vi "Drive Controller.vi"(8 "error in":errorcluster) -> ()   [LabVIEW 2023]
doc: "This VI executes continuously carrying out the current operation and responding to updates or new operation requests. It will often contain the timing or control code that is difficult to place directly in TeleOp. This VI generally opens all sensors and motors and isolates the rest of the robot code from knowing implementation details of how the operations are carried out."
uses:
  Drive Setpoints.ctl
  Drive Operations.ctl
  swerve-template/Type Definitions/Data/Robot Velocities.ctl
  <vilib>/Rock Robotics/WPI/ThirdParty/REV Robotics/REVLib/Typedef/Spark MAX Control Type.ctl
  80b923c8-6b82-42f9-a8cd-acddf0fa8107.vi
  Framework/Robot Global Data.vi
panel:
  in  "Drive Controller Diagnostics":T1(tab)
  out "Swerve Visualizer":cluster{dbl[], dbl[]}[](graph)
  out "Pod Comparisons (Diff -> Setpoint - Actual)":T2
  out "(Calibration) Steering Angles":T3
  out "Current\nCmd":string
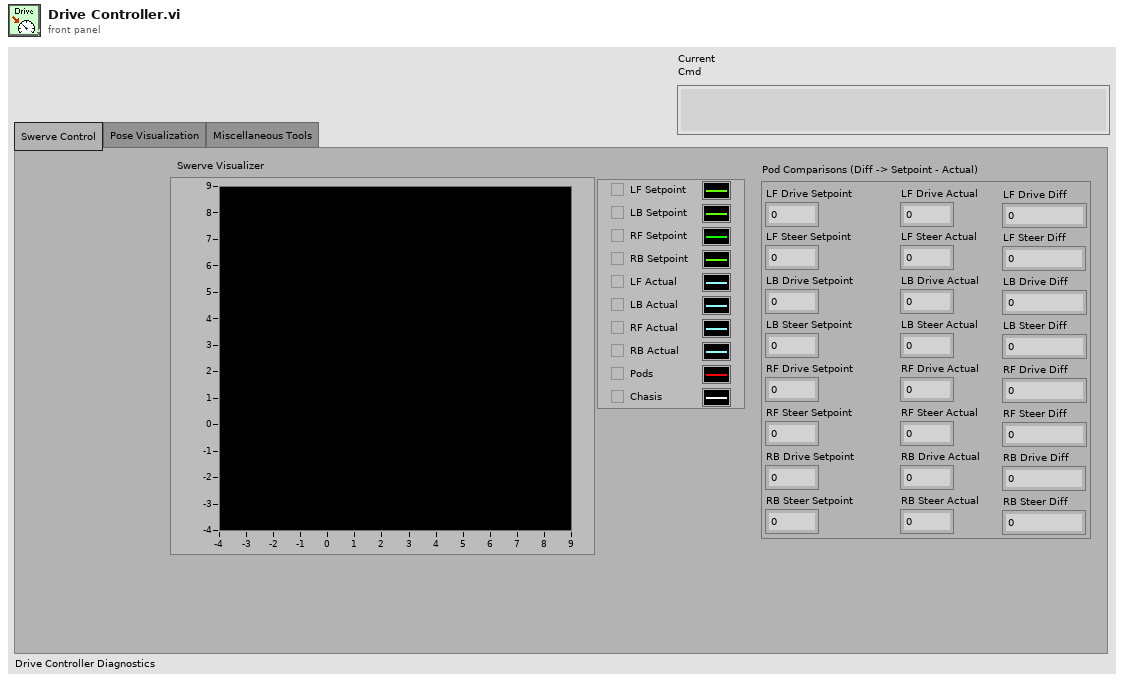
[diagram p1: front panel]
types:
  T1 = enum32{"Swerve Control", "Pose Visualization", "Miscellaneous Tools"}
  T2 = cluster{"LF Drive Setpoint":dbl, "LF Steer Setpoint":dbl, "LB Drive Setpoint":dbl, "LB Steer Setpoint":dbl, "RF Drive Setpoint":dbl, "RF Steer Setpoint":dbl, "RB Drive Setpoint":dbl, "RB Steer Setpoint":dbl, "LF Drive Actual":dbl, "LF Steer Actual":dbl, "LB Drive Actual":dbl, "LB Steer Actual":dbl, "RF Drive Actual":dbl, "RF Steer Actual":dbl, "RB Drive Actual":dbl, "RB Steer Actual":dbl, "LF Drive Diff":dbl, "LF Steer Diff":dbl, "LB Drive Diff":dbl, "LB Steer Diff":dbl, "RF Drive Diff":dbl, "RF Steer Diff":dbl, "RB Drive Diff":dbl, "RB Steer Diff":dbl}
  T3 = cluster{"Left Front":dbl, "Left Back":dbl, "Right Front":dbl, "Right Back":dbl}
  T4 = typedef "Drive Setpoints.ctl" = cluster{"Operation":T5, "Robot Velocities":T6, "Auto Data":cluster{"Auto Velocities":T6[], "Auto Positions":cluster{"x":dbl, "y":dbl, "th":dbl}[], "Auto Commands":cluster{dbl, "Command out":cluster{"Name":string, "vi reference":refnum<vi>, i32[], variant[]}}[], "Zero Velocity?":bool[]}}
  T5 = typedef "Drive Operations.ctl" = enum16{"Reserve", "Read Current", "Immediate", "Calibrate", "Auto"}
  T6 = typedef "Robot Velocities.ctl" = cluster{"X Velocity":dbl, "Y Velocity":dbl, "Rotational \nVelocity":dbl}
  T7 = typedef "(NEO-NEO-ThroughBore-Pigeon2) Swerve.ctl" = cluster{"Drive Motors (NEO)":T8, "Steer Motors (NEO)":T8, "Pigeon2":T14, "Radii (ft)":T16}
  T8 = typedef "(NEO & NEO 550) 4 Motor Set.ctl" = cluster{"Left Front":T9, "Left Back":T9, "Right Front":T9, "Right Back":T9}
  T9 = typedef "WPI_MotorControlDeviceRef.ctl" = cluster{"DeviceStatus":errorcluster, "Type":T10, "PWM":cluster{"PWM Channel":T11, "DeadBand":T12}, "CAN":cluster{"Device Number":u8, "SetOutput VI Ref":variant, "GetOutput VI Ref":variant, "Enable VI Ref":variant, "Disable VI Ref":variant, "Data":variant}, "Invert":bool, "DIO PWM":cluster{"PWM \"Enable\" Channel":T11, "DIOChannel":T13, "PWM Rate":dbl}}
  T10 = typedef "WPI_MotorControlType.ctl" = enum16{"PWM", "CAN", "DIO PWM"}
  T11 = typedef "FPGA_DIOPWMChannel.ctl" = enum8{"PWM 0", "PWM 1", "PWM 2", "PWM 3", "PWM 4", "PWM 5", "PWM 6", "PWM 7", "PWM 8", "PWM 9", "PWM MXP 0", "PWM MXP 1", "PWM MXP 2", "PWM MXP 3", "PWM MXP 4", "PWM MXP 5", "PWM MXP 6", "PWM MXP 7", "PWM MXP 8", "PWM MXP 9", "Invalid"}
  T12 = typedef "WPI_PWMDeadband.ctl" = cluster{"Name":string, "maxPositivePwm":i32, "minPositivePwm":i32, "centerPwm":i32, "maxNegativePwm":i32, "minNegativePwm":i32, "angularRange":u16}
  T13 = typedef "FPGA_DIOChannel.ctl" = enum8{"DIO 0", "DIO 1", "DIO 2", "DIO 3", "DIO 4", "DIO 5", "DIO 6", "DIO 7", "DIO 8", "DIO 9", "DIO MXP 0", "DIO MXP 1", "DIO MXP 2", "DIO MXP 3", "DIO MXP 4", "DIO MXP 5", "DIO MXP 6", "DIO MXP 7", "DIO MXP 8", "DIO MXP 9", "DIO MXP 10", "DIO MXP 11", "DIO MXP 12", "DIO MXP 13", "DIO MXP 14", "DIO MXP 15", "SPI Port CS1", "SPI Port CS2", "SPI Port CS3", "SPI Port MISO", "SPI Port MOSI", "Invalid"}
  T14 = typedef "CTRE_PigeonIMU_DeviceRef.ctl" = cluster{"DeviceStatus":errorcluster, "Device Number":u8, "Type":T15, "Device ID":u32, "Handle":u64, "UsageFrame":u32, "Library Path":path}
  T15 = typedef "CTRE_PigeonIMU_ConnectionType.ctl" = u32
  T16 = typedef "Pod Positions.ctl" = cluster{"Left Front Position":dbl[], "Left Back Position":dbl[], "Right Front Position":dbl[], "Right Back Position":dbl[]}
  T17 = typedef "Command Status Info.ctl" = cluster{"Name":string, "Status":T18, "notifier out":T19}
  T18 = typedef "Completion Status.ctl" = enum16{"Successful", "Aborted", "Incomplete"}
  T19 = typedef "Completion Notifier.ctl" = refnum<notifier>
  T20 = cluster{"SubSystem Data":T4, cluster{"Start Time (ms)":u32, "Iterations":i32}, cluster{"Command Info":T17, "Description":string, "Default Command":T4, "queue out":refnum<queue>, "Subsystem Name":string}}
  T21 = cluster{"Auto Velocities":T6[], "Auto Positions":cluster{"x":dbl, "y":dbl, "th":dbl}[], "Auto Commands":cluster{dbl, "Command out":cluster{"Name":string, "vi reference":refnum<vi>, i32[], variant[]}}[], "Zero Velocity?":bool[]}
  T22 = typedef "Pod Setpoints.ctl" = cluster{"Left Front":cluster{"Velocity":dbl, "Theta":dbl}, "Left Back":cluster{"Velocity":dbl, "Theta":dbl}, "Right Front":cluster{"Velocity":dbl, "Theta":dbl}, "Right Back":cluster{"Velocity":dbl, "Theta":dbl}}
  T23 = typedef "Spark MAX Control Type.ctl" = enum16{"Percent VBus", "Voltage", "Velocity", "Position", "Smart Motion", "Current", "Smart Velocity", "MAXMotion Position", "MAXMotion Velocity"}
  T24 = cluster{"SubSystem Data":T4, cluster{"Start Time (ms)":u32, "Iterations":i32}, "Default Command Arguments":cluster{"Command Info":T17, "Description":string, "Default Command":T4, "queue out":refnum<queue>, "Subsystem Name":string}}
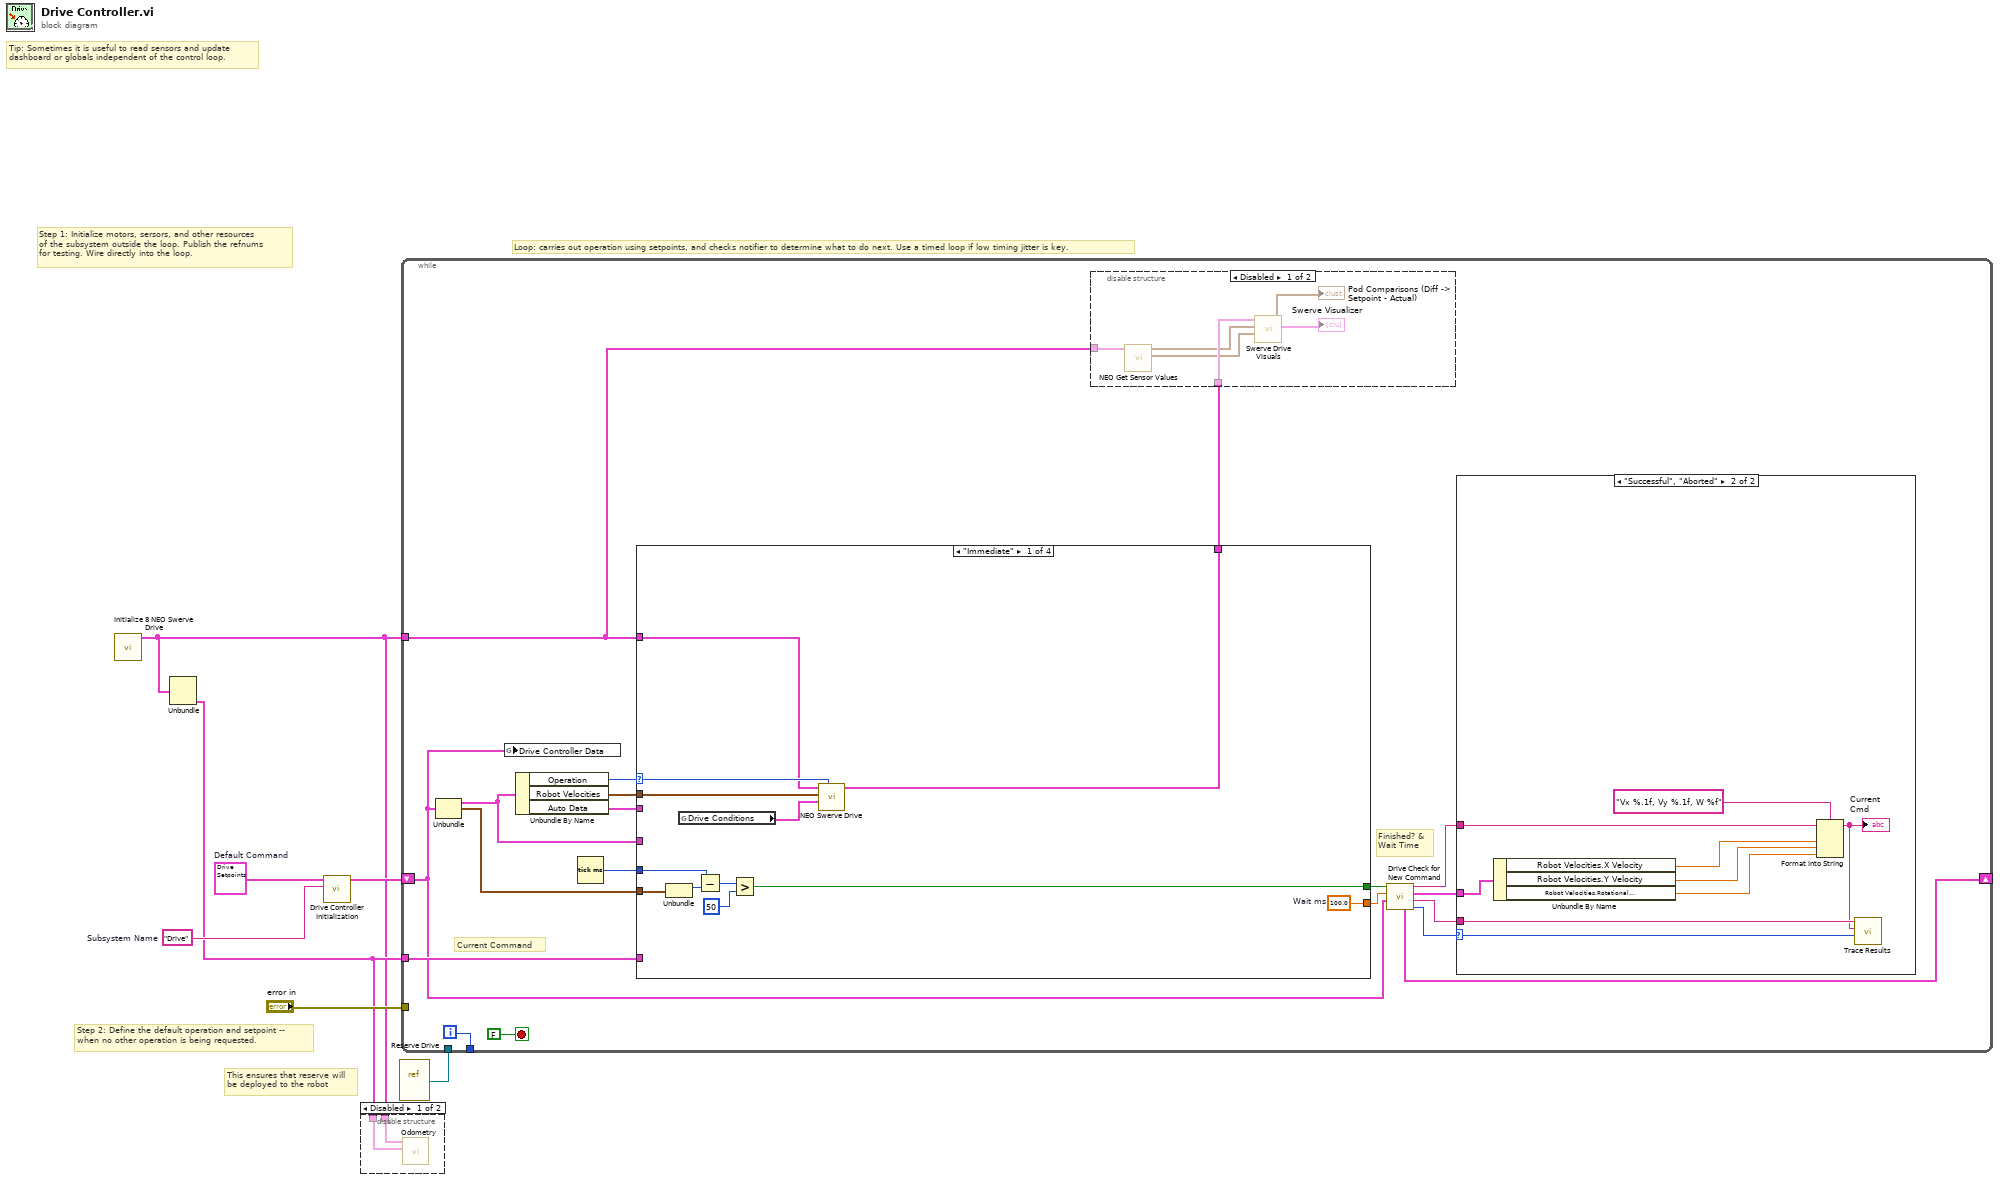
[diagram p0: block diagram]
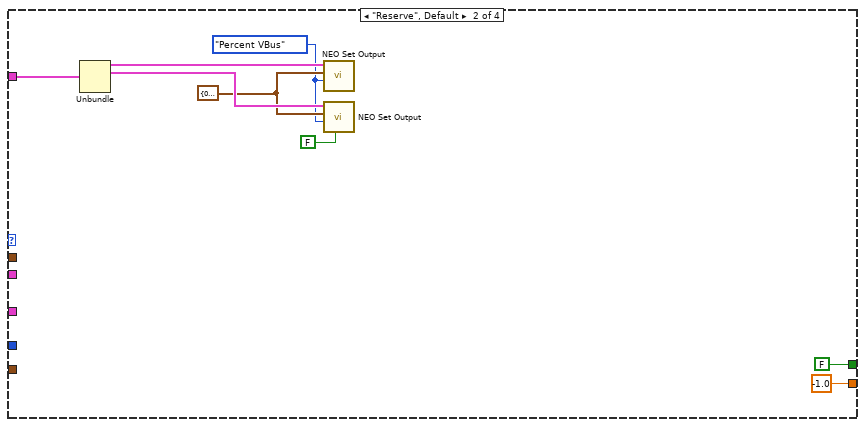
[diagram p4: hidden frame]
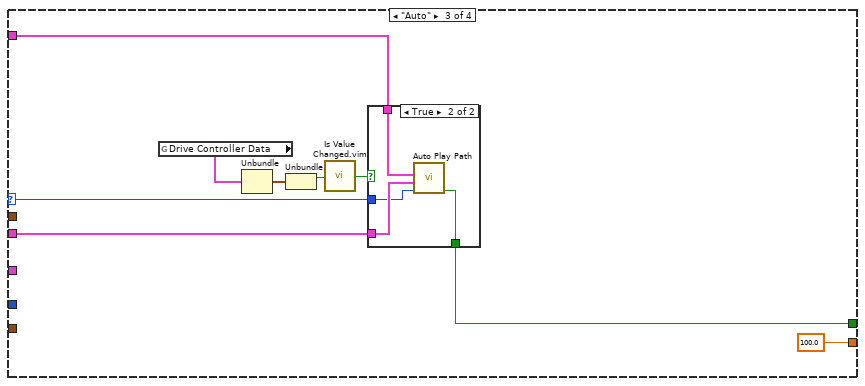
[diagram p5: hidden frame]
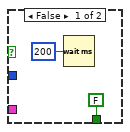
[diagram p6: hidden frame]
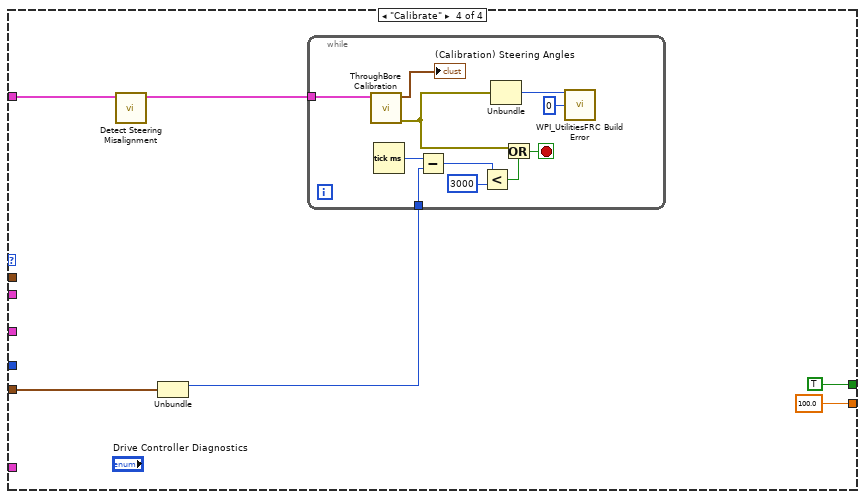
[diagram p7: hidden frame]
diagram:
  w3 = T4 {"Operation"=enum."Reserve", "Robot Velocities"={"X Velocity"=0.0, "Y Velocity"=0.0, "Rotational \nVelocity"=0.0}, "Auto Data"={"Auto Velocities"=[], "Auto Positions"=[], "Auto Commands"=[], "Zero Velocity?"=[]}}  # Default Command
  w7 = "Drive"  # Subsystem Name
  # "This ensures that reserve will\nbe deployed to the robot"
  # "Step 2: Define the default operation and setpoint --\nwhen no other operation is being requested."
  # "Step 1: Initialize motors, sersors, and other resources\nof the subsystem outside the loop. Publish the refnums\nfor testing. Wire directly into the loop."
  # "Loop: carries out operation using setpoints, and checks notifier to determine what to do next. Use a timed loop if low timing jitter is key."
  # "Tip: Sometimes it is useful to read sensors and update\ndashboard or globals independent of the control loop."
  n1 = call "Initialize 8 NEO Swerve Drive.vi"() -> ("Motors"=w1:T7)  [unwired: 10 in, 1 out]
  n2 = Unbundle(w1) -> ("Radii (ft)"=w2:T16)  [unwired: 3 out]
  n3 = call "Drive Controller Initialization.vi"("Subsystem Name"=w7, "Default Command"=w3) -> ("Current Command"=w5:T20)  [unwired: 9 in]
  n4 = disable-structure shown="Disabled" {
    disable-tunnel: w2 -> [w9 _]
    disable-tunnel: w1 -> [w8 _]
    frame Disabled {
      n5 = call "Odometry.vi"("Radii (ft)"=w9, "Motors"=w8) -> ()  [unwired: 10 in]
    }
    frame Enabled {
    }
  }
  n6 = vi-ref "Reserve Drive.vi"() -> (w4:refnum<vi>)
  n7 = while {
    shift-right: [w20] -> _
    shift-left: w5 -> [w10]
    tunnel: [w27] -> _
    tunnel: "error in" -> [_]
    tunnel: w4 -> [_]
    tunnel: w1 -> [w18]
    tunnel: w2 -> [w21]
    i -> [w27]
    stop <- FALSE stop-if-true
    # "Current Command"
    # "Finished? &\nWait Time"
    n8 = Unbundle(w10) -> ("SubSystem Data"=w13:T4, w11:cluster{"Start Time (ms)":u32, "Iterations":i32})  [unwired: 1 out]
    n9 = global write "Robot Global Data.vi" "Drive Controller Data"(w10) -> ()
    n10 = Unbundle By Name(w13) -> ("Operation"=w16:T5, "Robot Velocities"=w22:T6, "Auto Data"=w17:T21)
    n11 = Tick Count (ms)() -> (millisecond timer value=w12:u32)
    n12 = case shown="\"Immediate\"" w16 {
      selector: w16 -> [w38 _ w56 _]
      tunnel: [w46 -1.0 ("Infinite") 100.0 100.0 ("Infinite")] -> w26
      tunnel: [w41 FALSE ("ignore previous (F)") w55 TRUE ("ignore previous (F)")] -> w25
      tunnel: w11 -> [w45 _ _ w73]
      tunnel: w12 -> [w40 _ _ _]
      tunnel: w22 -> [w37 _ _ _]
      tunnel: w18 -> [w35 w52 w63 w71]
      tunnel: w21 -> [_ _ _ _]
      tunnel: [w39 _ _ _] -> w19
      tunnel: w13 -> [_ _ _ _]
      tunnel: w17 -> [_ _ w61 _]
      frame "Immediate" {
        w46 = 100.0  # Wait ms
        n13 = Unbundle(w45) -> ("Start Time (ms)"=w44:u32)  [unwired: 1 out]
        n14 = global read "Robot Global Data.vi" "Drive Conditions"() -> (w36:cluster{"Field Centric":bool})
        n15 = Subtract(x=w40, y=w44) -> (x-y=w43:u32)
        n16 = Greater?(x=w43, y=u32 50) -> (0:w41:bool)
        n17 = call "NEO Swerve Drive.vi"("Operation"=w38, "Drive Conditions"=w36, "Robot Velocities"=w37, "Swerve Drive"=w35) -> ("Pod Setpoints (ft/s and deg)"=w39:T22)  [unwired: 7 in]
      }
      frame "Reserve", Default {
        w47 = Spark_MAX_Control_Type."Percent VBus" ("Reserve Control Mode")
        w48 = T3 {"Left Front"=0.0, "Left Back"=0.0, "Right Front"=0.0, "Right Back"=0.0} ("Setpoints")
        n18 = Unbundle(w52) -> ("Drive Motors (NEO)"=w51:T8, "Steer Motors (NEO)"=w50:T8)  [unwired: 2 out]
        n19 = call "NEO Set Output.vi"("Control Mode"=w47, "Setpoints"=w48, "Motors"=w51) -> ()  [unwired: 9 in]
        n20 = call "NEO Set Output.vi"("Add Angle Offsets?"=FALSE, "Control Mode"=w47, "Setpoints"=w48, "Motors"=w50) -> ()  [unwired: 8 in]
      }
      frame "Auto" {
        n21 = global read "Robot Global Data.vi" "Drive Controller Data"() -> (w60:T20)
        n22 = Unbundle(w60) -> (w59:cluster{"Start Time (ms)":u32, "Iterations":i32})  [unwired: 2 out]
        n23 = Unbundle(w59) -> ("Start Time (ms)"=w58:u32)  [unwired: 1 out]
        n24 = call "Is Value Changed.vim"("value"=w58) -> ("changed or first call?"=w57:bool)
        n25 = case shown="True" w57 {
          tunnel: w61 -> [_ w68]
          tunnel: w63 -> [_ w69]
          tunnel: w56 -> [_ w67]
          tunnel: [FALSE ("Auto Done?") w66] -> w55
          frame False {
            n26 = Wait (ms)(milliseconds to wait=u32 200) -> ()  [unwired: 1 out]
          }
          frame True {
            n27 = call "Auto Play Path.vi"("Operation"=w67, "Auto Data"=w68, "Motors"=w69) -> ("Auto Done?"=w66:bool)  [unwired: 8 in]
          }
        }
      }
      frame "Calibrate" {
        n28 = call "Detect Steering Misalignment.vi"("Motors In"=w71) -> ("Motors Out"=w70:T7)  [unwired: 10 in]
        n29 = Unbundle(w73) -> ("Start Time (ms)"=w72:u32)  [unwired: 1 out]
        n30 = while {
          tunnel: w70 -> [w80]
          tunnel: w72 -> [w85]
          stop <- w86 stop-if-true
          n31 = call "ThroughBore Calibration.vi"("Motors"=w80) -> ("error out"=w77:errorcluster, "Steering Angles"=→"(Calibration) Steering Angles":cluster{"LF":dbl, "LB":dbl, "RF":dbl, "RB":dbl})  [unwired: 9 in]
          n32 = Tick Count (ms)() -> (millisecond timer value=w84:u32)
          n33 = Subtract(x=w84, y=w85) -> (x-y=w83:u32)
          n34 = Less?(x=w83, y=u32 3000) -> (x < y?=w81:bool)
          n35 = Unbundle(w77) -> ("code"=w76:i32)  [unwired: 2 out]
          n36 = Or(x=w77, y=w81) -> (x .or. y?=w86:bool)
          n37 = call <vilib>:"WPI_UtilitiesFRC Build Error.vi"("error code"=w76, "chain levels to remove (1)"=0) -> ()  [unwired: 3 in, 11 out]
        }
      }
    }
    n38 = disable-structure shown="Disabled" {
      disable-tunnel: w19 -> [w32 _]
      disable-tunnel: w18 -> [w29 _]
      frame Disabled {
        n39 = call "NEO Get Sensor Values.vi"("Swerve Motors"=w29) -> ("Steer Angles (degrees)"=w30:T3, "Drive Velocities (ft/s)"=w31:T3)  [unwired: 9 in]
        n40 = call "Swerve Drive Visuals.vi"("Steer Angles (degrees)"=w30, "Drive Velocities (ft/s)"=w31, "Pod Setpoints (ft/s and deg)"=w32) -> ("Swerve Visualizer"=→"Swerve Visualizer":cluster{dbl[], dbl[]}[], "Pod Comparisons (Diff -> Setpoint - Actual)"=→"Pod Comparisons (Diff -> Setpoint - Actual)":T2)  [unwired: 7 in]
      }
      frame Enabled {
      }
    }
    n41 = call "Drive Check for New Command.vi"("input cluster"=w10, "Wait time (ms)"=w26, "Finished?"=w25) -> ("Completion"=w15:T18, "Subsystem Name"=w23:string, "Current Command"=w14:T4, "Initial Trace String"=w24:string, "Next Command"=w20:T24)  [unwired: 4 in]
    n42 = case shown="\"Successful\", \"Aborted\"" w15 {
      selector: w15 -> [_ w87]
      tunnel: w24 -> [_ w94]
      tunnel: w14 -> [_ w95]
      tunnel: w23 -> [_ w93]
      frame "Incomplete", Default {
        # "Continuing current command"
      }
      frame "Successful", "Aborted" {
        # "Report and setup for next command"
        n43 = Unbundle By Name(w95) -> ("Robot Velocities.X Velocity"=w91:dbl, "Robot Velocities.Y Velocity"=w92:dbl, "Robot Velocities.Rotational \nVelocity"=w88:dbl)
        n44 = Format Into String(format string="Vx %.1f, Vy %.1f, W %f", initial string=w94, w91, w92, w88) -> (resulting string=w89:string)  [unwired: 1 in, 1 out]
        "Current\nCmd" <- w89
        n45 = call <vilib>:"Trace Results.vi"("Status of previous command"=w87, "Description"=w89, "Subsystem"=w93) -> ()  [unwired: 9 in]
      }
    }
  }
